vi "ep_Check Speed Nameplate (1 Motor).vi"(7 "check? (F)":bool, 8 "error in (no error)":errorcluster, 11 "nameplate information":T1) -> (0 "error out":errorcluster)   [LabVIEW 2014, in "NI_EP_Motor Monitoring.lvlib"]
uses:
  <vilib>/addons/Electrical Power/Motor Monitoring/NI_EP_Motor Monitoring.lvlib
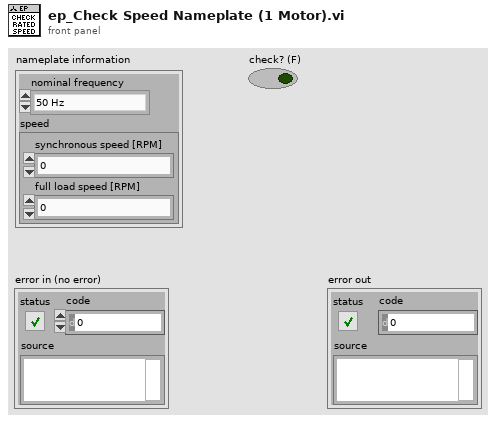
[diagram p1: front panel]
types:
  T1 = cluster{"nominal frequency":enum16{"50 Hz", "60 Hz"}, "speed":cluster{"synchronous speed [RPM]":dbl, "full load speed [RPM]":dbl}}
  T2 = cluster{"synchronous speed [RPM]":dbl, "full load speed [RPM]":dbl}
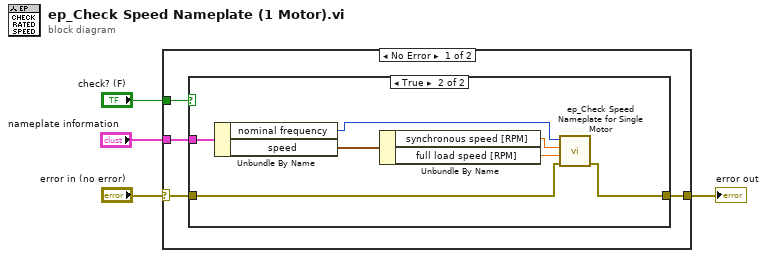
[diagram p0: block diagram]
diagram:
  n1 = case shown="No Error" "error in (no error)" {
    selector: "error in (no error)" -> [w6 w17]
    tunnel: [w7 w17] -> w3
    tunnel: "nameplate information" -> [w8 _]
    tunnel: "check? (F)" -> [w5 _]
    frame No Error {
      n2 = case shown="True" w5 {
        tunnel: w8 -> [_ w14]
        tunnel: [w9 w16] -> w7
        tunnel: w6 -> [w9 w15]
        frame False {
        }
        frame True {
          n3 = Unbundle By Name(w14) -> ("nominal frequency"=w12:enum16{"50 Hz", "60 Hz"}, "speed"=w13:T2)
          n4 = Unbundle By Name(w13) -> ("synchronous speed [RPM]"=w10:dbl, "full load speed [RPM]"=w11:dbl)
          n5 = call <vilib>:"ep_Check Speed Nameplate for Single Motor.vi"("error in (no error)"=w15, "full load speed [RPM]"=w11, "synchronous speed [RPM]"=w10, "nominal frequency"=w12) -> ("error out"=w16:errorcluster)  [unwired: 7 in]
        }
      }
    }
    frame Error {
    }
  }
  "error out" <- w3
